vi "average.vi"(8 "Numeric 2":dbl, 11 "Numeric":dbl) -> (1 "Numeric 3":dbl)   [LabVIEW 2015]
panel:
  in  "stop":bool
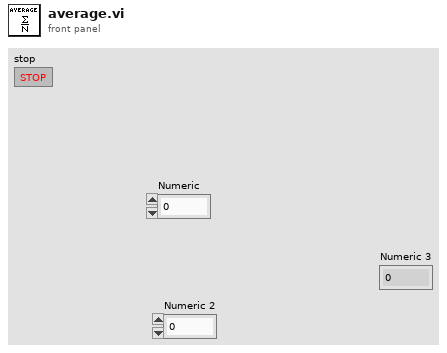
[diagram p1: front panel]
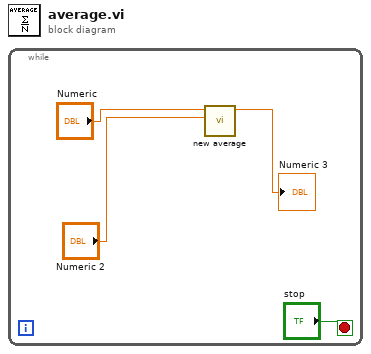
[diagram p0: block diagram]
diagram:
  n1 = while {
    stop <- "stop" stop-if-true
    n2 = call "new average.vi"("Numeric 3"="Numeric 2", "Numeric in"="Numeric") -> ("Numeric out"=→"Numeric 3":dbl)  [unwired: 9 in]
  }
